vi "niSwitch Get gRPC Location.vi"(8 "error in":errorcluster) -> (0 "error out":errorcluster, 2 "port":u32, 3 "address":string)   [LabVIEW 2021, in "Session Management niSwitch.lvlib" / "Session Factory.lvclass"]
doc: "Get the address and port location of NI gRPC Device Server."
uses:
  Session Factory.lvclass
  <vilib>/gRPC/Generated APIs/ni/measurementlink/discovery/v1/RPC Messages/ni_measurementlink_discovery_v1_ResolveServiceRequest.ctl
  Session Factory.lvclass/Session Factory.ctl
  <vilib>/Plug-In SDKs/Clients/Discovery V1/NI Discovery V1 Client.lvlib
  <vilib>/gRPC/Generated APIs/ni/measurementlink/discovery/v1/ni.measurementlink.discovery.v1.api.lvlib
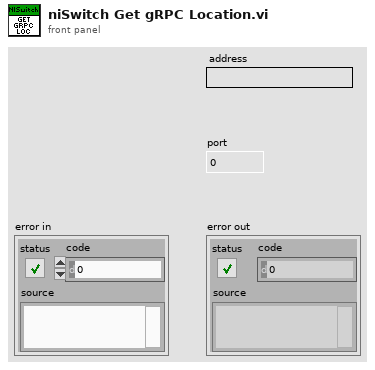
[diagram p1: front panel]
types:
  T1 = typedef "ni.measurementlink.discovery.v1.api.lvlib/ni_measurementlink_discovery_v1_ResolveServiceRequest.ctl" = cluster{"provided_interface":string, "service_class":string, "deployment_target":string, "version":string}
  T2 = typedef "ni.measurementlink.discovery.v1.api.lvlib/ni_measurementlink_discovery_v1_ServiceLocation.ctl" = cluster{"location":string, "insecure_port":string, "ssl_authenticated_port":string}
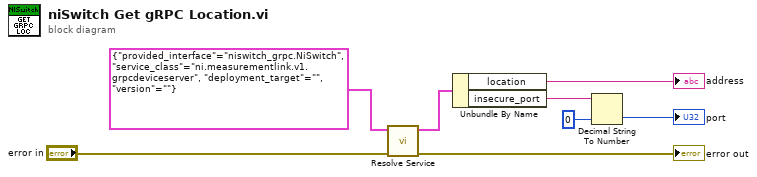
[diagram p0: block diagram]
diagram:
  n1 = call <vilib>:"Resolve Service.vi"("error in"="error in", "request data"=T1 {"provided_interface"="niswitch_grpc.NiSwitch", "service_class"="ni.measurementlink.v1.grpcdeviceserver", "deployment_target"="", "version"=""}) -> ("error out"=→"error out":errorcluster, "response data"=w1:T2)  [unwired: 8 in]
  n2 = Unbundle By Name(w1) -> ("location"=→"address":string, "insecure_port"=w6:string)
  n3 = Decimal String To Number(string=w6, default (0L)=u32 0 ("default (0 I32)")) -> (number=→"port":u32)  [unwired: 1 in, 1 out]
